vi "Test Unnamed Clusters to JSON Arrays.vi"() -> ()   [LabVIEW 2013]
uses:
  JSONtext.lvlib
panel:
  out "<JSON>":string
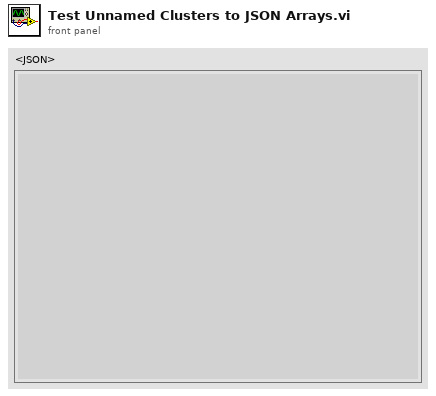
[diagram p1: front panel]
types:
  T1 = cluster{cluster{string, "<JSON>":string, i32}, "<JSON>":string, "<JSON>":string}
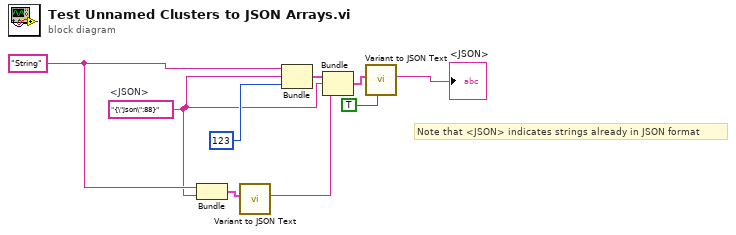
[diagram p0: block diagram]
diagram:
  w4 = "{\"Json\":88}"  # <JSON>
  w5 = "String"
  # "Note that <JSON> indicates strings already in JSON format"
  n1 = Bundle(w5, "<JSON>"=w4) -> (w3:cluster{string, "<JSON>":string})  [unwired: 1 in]
  n2 = call "Variant to JSON Text.vi"("Variant"=w3) -> ("<JSON>"=w2:string)  [unwired: 9 in, 1 out]
  n3 = Bundle(w5, "<JSON>"=w4, 123) -> (w8:cluster{string, "<JSON>":string, i32})  [unwired: 1 in]
  n4 = Bundle(w8, "<JSON>"=w4, "<JSON>"=w2) -> (w7:T1)  [unwired: 1 in]
  n5 = call "Variant to JSON Text.vi"("Pretty Print?"=TRUE, "Variant"=w7) -> ("<JSON>"=→"<JSON>":string)  [unwired: 8 in, 1 out]
